vi "server hello world.vi"() -> ()   [LabVIEW 2016]
uses:
  lvlibtls/server/lvlibretls server listener.lvclass
  C:/Users/IEUser/Desktop/lvlibtls/lvlibtls/context parent/lvlibretls configurable context.lvclass
  lvlibtls/context parent/lvlibretls configurable context.lvclass
  lvlibtls/socket connection/lvlibretls connection.lvclass
panel:
  out "error out":errorcluster
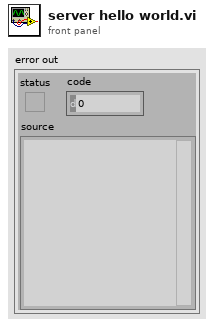
[diagram p1: front panel]
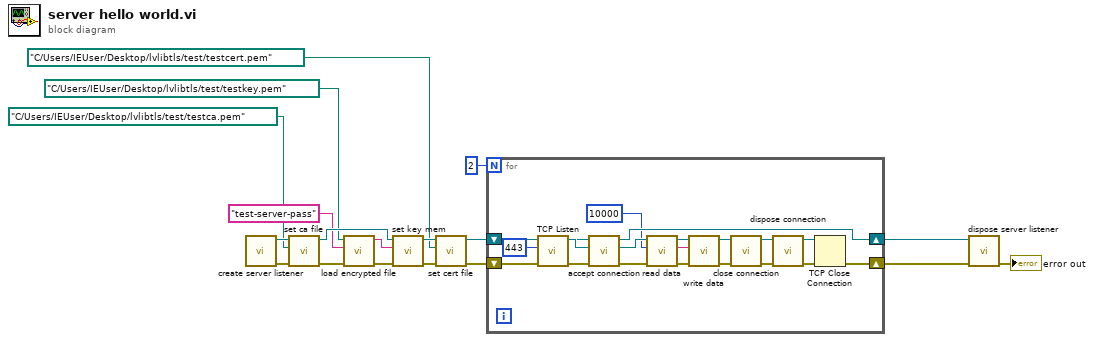
[diagram p0: block diagram]
diagram:
  n1 = call "create server listener.vi"() -> ("error out"=w17:errorcluster, "lvlibretls server listener out"=w18:refnum<class "lvlibretls server listener.lvclass">)  [unwired: 10 in]
  n2 = call "set ca file.vi"("error in"=w17, "ca file"=path "C:/Users/IEUser/Desktop/lvlibtls/test/testca.pem", "lvlibretls configurable context in"=w18) -> ("error out"=w8:errorcluster, "lvlibretls configurable context out"=w7:refnum<class "lvlibretls server listener.lvclass">)  [unwired: 7 in]
  n3 = call "load encrypted file.vi"("error in"=w8, "password"="test-server-pass", "Path"=path "C:/Users/IEUser/Desktop/lvlibtls/test/testkey.pem" ("key file")) -> ("error out"=w11:errorcluster, "data"=w12:string)  [unwired: 7 in]
  n4 = call "set key mem.vi"("error in"=w11, "key file"=w12, "lvlibretls configurable context in"=w7) -> ("error out"=w9:errorcluster, "lvlibretls configurable context out"=w10:refnum<class "lvlibretls server listener.lvclass">)  [unwired: 7 in]
  n5 = call "set cert file.vi"("error in"=w9, "cert file"=path "C:/Users/IEUser/Desktop/lvlibtls/test/testcert.pem" ("ca file"), "lvlibretls configurable context in"=w10) -> ("error out"=w5:errorcluster, "lvlibretls configurable context out"=w6:refnum<class "lvlibretls server listener.lvclass">)  [unwired: 7 in]
  n6 = for {
    N: 2 -> [_]
    shift-right: [w29] -> w14
    shift-left: w6 -> [w20]
    shift-right: [w31] -> w15
    shift-left: w5 -> [w19]
    n7 = call <vilib>:"TCP Listen.vi"("error in (no error)"=w19, "port"=u16 443) -> ("error out"=w35:errorcluster, "connection ID"=w36:refnum<k5>)  [unwired: 5 in, 3 out]
    n8 = call "accept connection.vi"("error in"=w35, "connection ID"=w36, "lvlibretls server listener in"=w20) -> ("error out"=w27:errorcluster, "lvlibretls connection"=w28:refnum<class "lvlibretls connection.lvclass">, "lvlibretls server listener out"=w29:refnum<class "lvlibretls server listener.lvclass">)  [unwired: 6 in]
    n9 = call "read data.vi"("error in"=w27, "max size"=10000, "lvlibretls connection in"=w28) -> ("error out"=w25:errorcluster, "data"=w22:string, "lvlibretls connection out"=w26:refnum<class "lvlibretls connection.lvclass">)  [unwired: 6 in]
    n10 = call "write data.vi"("error in"=w25, "data"=w22, "lvlibretls connection in"=w26) -> ("error out"=w23:errorcluster, "lvlibretls connection out"=w24:refnum<class "lvlibretls connection.lvclass">)  [unwired: 7 in]
    n11 = call "close connection.vi"("error in"=w23, "lvlibretls connection in"=w24) -> ("error out"=w33:errorcluster, "lvlibretls connection out"=w34:refnum<class "lvlibretls connection.lvclass">)  [unwired: 8 in]
    n12 = call "dispose connection.vi"("error in"=w33, "lvlibretls connection in"=w34) -> ("error out"=w32:errorcluster, "connection"=w30:refnum<k5>)  [unwired: 8 in]
    n13 = TCP Close Connection(connection ID=w30, error in (no error)=w32) -> (error out=w31:errorcluster)  [unwired: 1 in, 1 out]
  }
  n14 = call "dispose server listener.vi"("error in"=w15, "lvlibretls server listener in"=w14) -> ("error out"=→"error out":errorcluster)  [unwired: 9 in]
